vi "convert_exposure_time.vi"(9 "Exposure (s)":dbl, 10 "Preview binning":dbl, 11 "Capture binning":dbl) -> (3 "Converted exposure (s)":dbl)   [LabVIEW 2011]
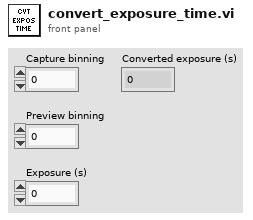
[diagram p1: front panel]
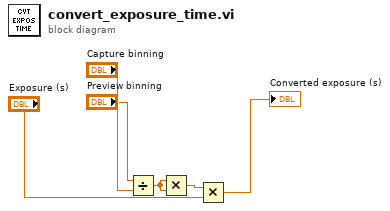
[diagram p0: block diagram]
diagram:
  n1 = Divide(x="Preview binning", y="Capture binning") -> (x/y=w1:dbl)
  n2 = Multiply(x=w1, y=w1) -> (x*y=w2:dbl)
  n3 = Multiply(x=w2, y="Exposure (s)") -> (x*y=→"Converted exposure (s)":dbl)
